vi "Add_task_name.vi"(8 "error in (no error)":errorcluster, 10 "new name of task":string, 11 "DAQmxTaksContainer_General in":refnum<class "DAQmxTaksContainer_General.lvclass">) -> (0 "error out":errorcluster, 3 "DAQmxTaksContainer_General out":refnum<class "DAQmxTaksContainer_General.lvclass">)   [LabVIEW 2015, in "DAQmxTaksContainer_General.lvclass"]
uses:
  DAQmxTaksContainer_General.lvclass
  DAQmxTaksContainer_General.lvclass/DAQmxTaksContainer_General.ctl
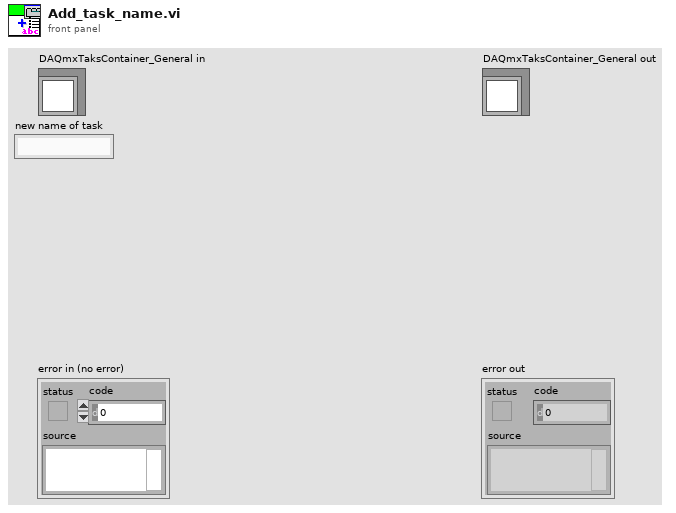
[diagram p1: front panel]
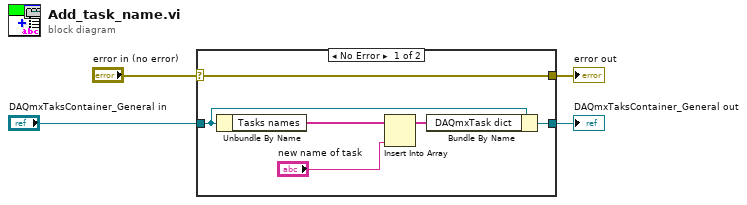
[diagram p0: block diagram]
diagram:
  n1 = case shown="No Error" "error in (no error)" {
    selector: "error in (no error)" -> [w10 w12]
    tunnel: [w10 w12] -> w3
    tunnel: [w7 w11] -> w1
    tunnel: "DAQmxTaksContainer_General in" -> [w8 w11]
    frame No Error {
      n2 = Unbundle By Name(w8) -> ("Tasks names"=w9:string[])
      n3 = Insert Into Array(array=w9, new element="new name of task") -> (w6:string[])  [unwired: 1 in]
      n4 = Bundle By Name(cluster=w8, "DAQmxTask dict"=w6) -> (w7:refnum<class "DAQmxTaksContainer_General.lvclass">)
    }
    frame Error {
    }
  }
  "error out" <- w3
  "DAQmxTaksContainer_General out" <- w1
